vi "Replace Float Array Subset.vi"(1 "New elements":dbl[](array[numeric]) format="%.2f", 2 "Index (0)":i32, 4 "Input array":dbl[](array[numeric]) format="%.2f") -> (0 "Output array":dbl[](array[numeric]) format="%.2f")   [LabVIEW 2017]
doc: "Anritsu LabVIEW Toolkit\n\nA LabVIEW-5-compatible implementation of Replace Array Subset. Replaces a group of elements in a 1-D array with new values.\n\nINPUTS\n Input array - the array whose values will be overwritten.\n Index - location of the first value to be overwritten.\n New elements - values to be written into the array.\n\nOUTPUTS\n Output array - array with the new values."
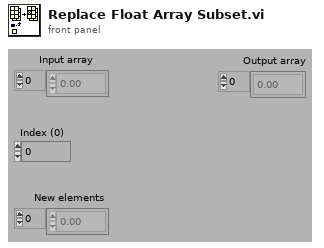
[diagram p1: front panel]
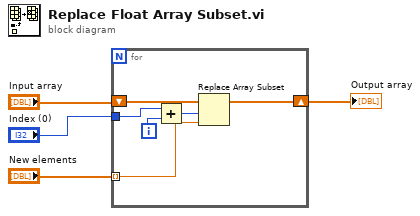
[diagram p0: block diagram]
diagram:
  n1 = for {
    tunnel: "New elements" -> [w6] mode=indexing
    tunnel: "Index (0)" -> [w9]
    shift-right: [w7] -> w1
    shift-left: "Input array" -> [w8]
    i -> [w10]
    n2 = Add(x=w9, y=w10) -> (x+y=w5:i32)
    n3 = Replace Array Subset(array=w8, new element=w6, index=w5) -> (w7:dbl[])
  }
  "Output array" <- w1
